vi "AB_1200_1300_Project_App_Info.vi"(6 "dataForPrevious in":T1, 7 "action":T2, 8 "error in (no error)":errorcluster, 10 "applicationInfo in":T3, 11 "Object In":T4) -> (0 "error out":errorcluster, 2 "Application info":T3, 3 "Object Out":T4, 4 "dataFromPrevious":T1)   [LabVIEW 2020]
uses:
  <resource>/Framework/Providers/API/ItemRef.ctl
  <vilib>/AppBuilder/RW_Project/AB_RW_Project_PropBag_Action.ctl
  <vilib>/AppBuilder/RW_Project/AB_RW_Project_App_Data_for_Previous.ctl
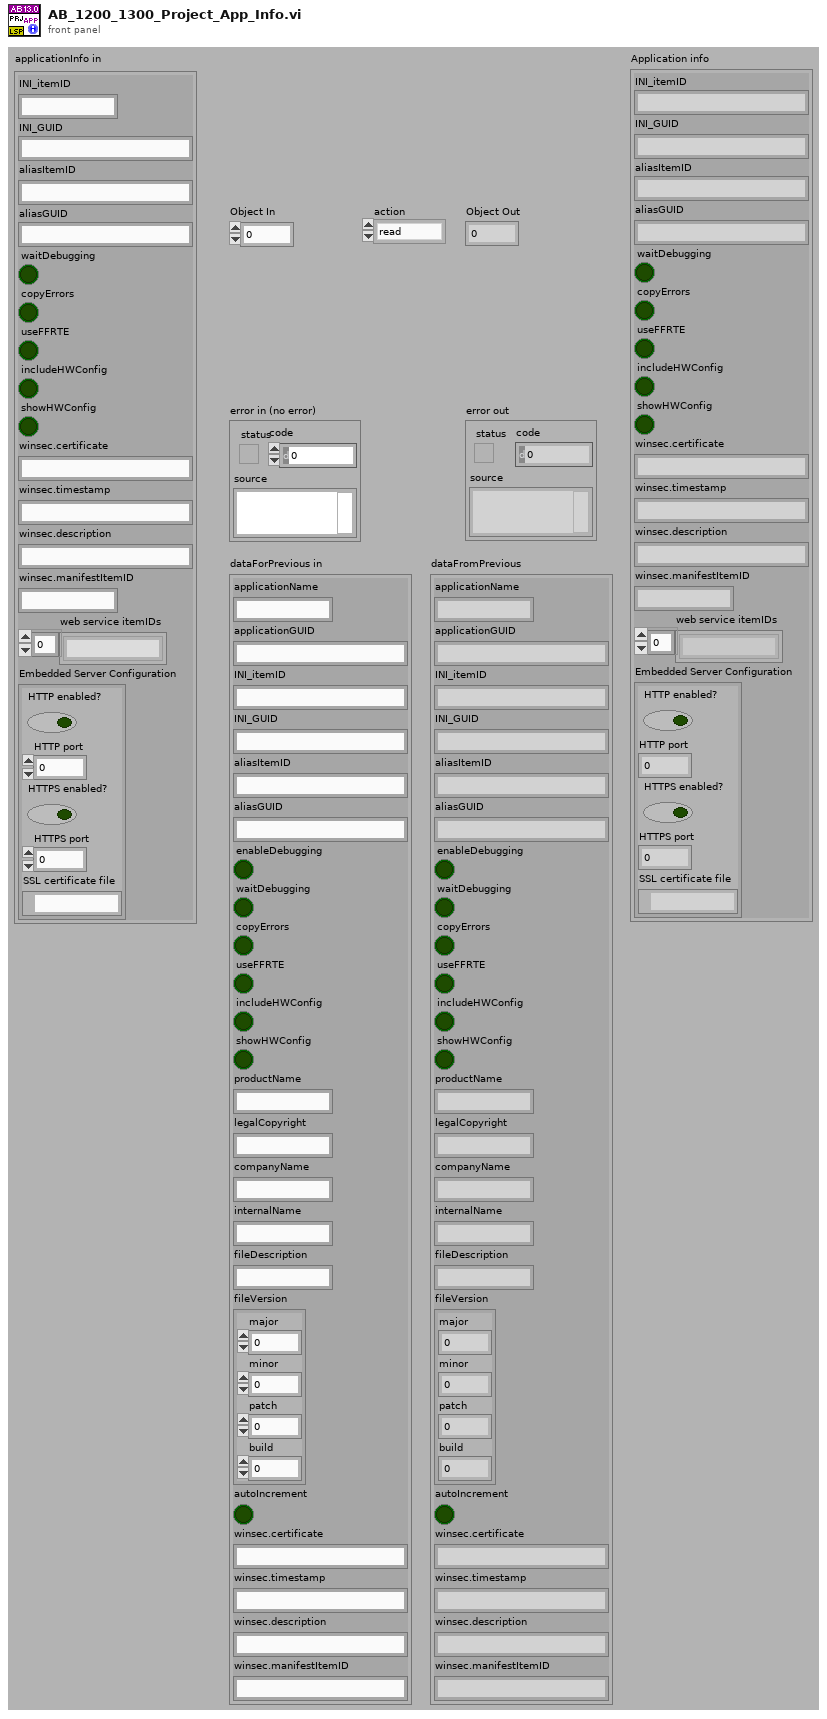
[diagram p1: front panel]
types:
  T1 = typedef "AB_RW_Project_App_Data_for_Previous.ctl" = cluster{"applicationName":string, "applicationGUID":string, "INI_itemID":string, "INI_GUID":string, "aliasItemID":string, "aliasGUID":string, "enableDebugging":bool, "waitDebugging":bool, "copyErrors":bool, "useFFRTE":bool, "includeHWConfig":bool, "showHWConfig":bool, "productName":string, "legalCopyright":string, "companyName":string, "internalName":string, "fileDescription":string, "fileVersion":cluster{"major":u16, "minor":u16, "patch":u16, "build":u16}, "autoIncrement":bool, "winsec.certificate":string, "winsec.timestamp":string, "winsec.description":string, "winsec.manifestItemID":string}
  T2 = typedef "AB_RW_Project_PropBag_Action.ctl" = enum16{"read", "write", "clear", "readPrevious", "writePrevious", "clearPrevious"}
  T3 = cluster{"INI_itemID":string, "INI_GUID":string, "aliasItemID":string, "aliasGUID":string, "waitDebugging":bool, "copyErrors":bool, "useFFRTE":bool, "includeHWConfig":bool, "showHWConfig":bool, "winsec.certificate":string, "winsec.timestamp":string, "winsec.description":string, "winsec.manifestItemID":string, "web service itemIDs":string[], "Embedded Server Configuration":cluster{"HTTP enabled?":bool, "HTTP port":i32, "HTTPS enabled?":bool, "HTTPS port":i32, "SSL certificate file":path}}
  T4 = typedef "ItemRef.ctl" = u64
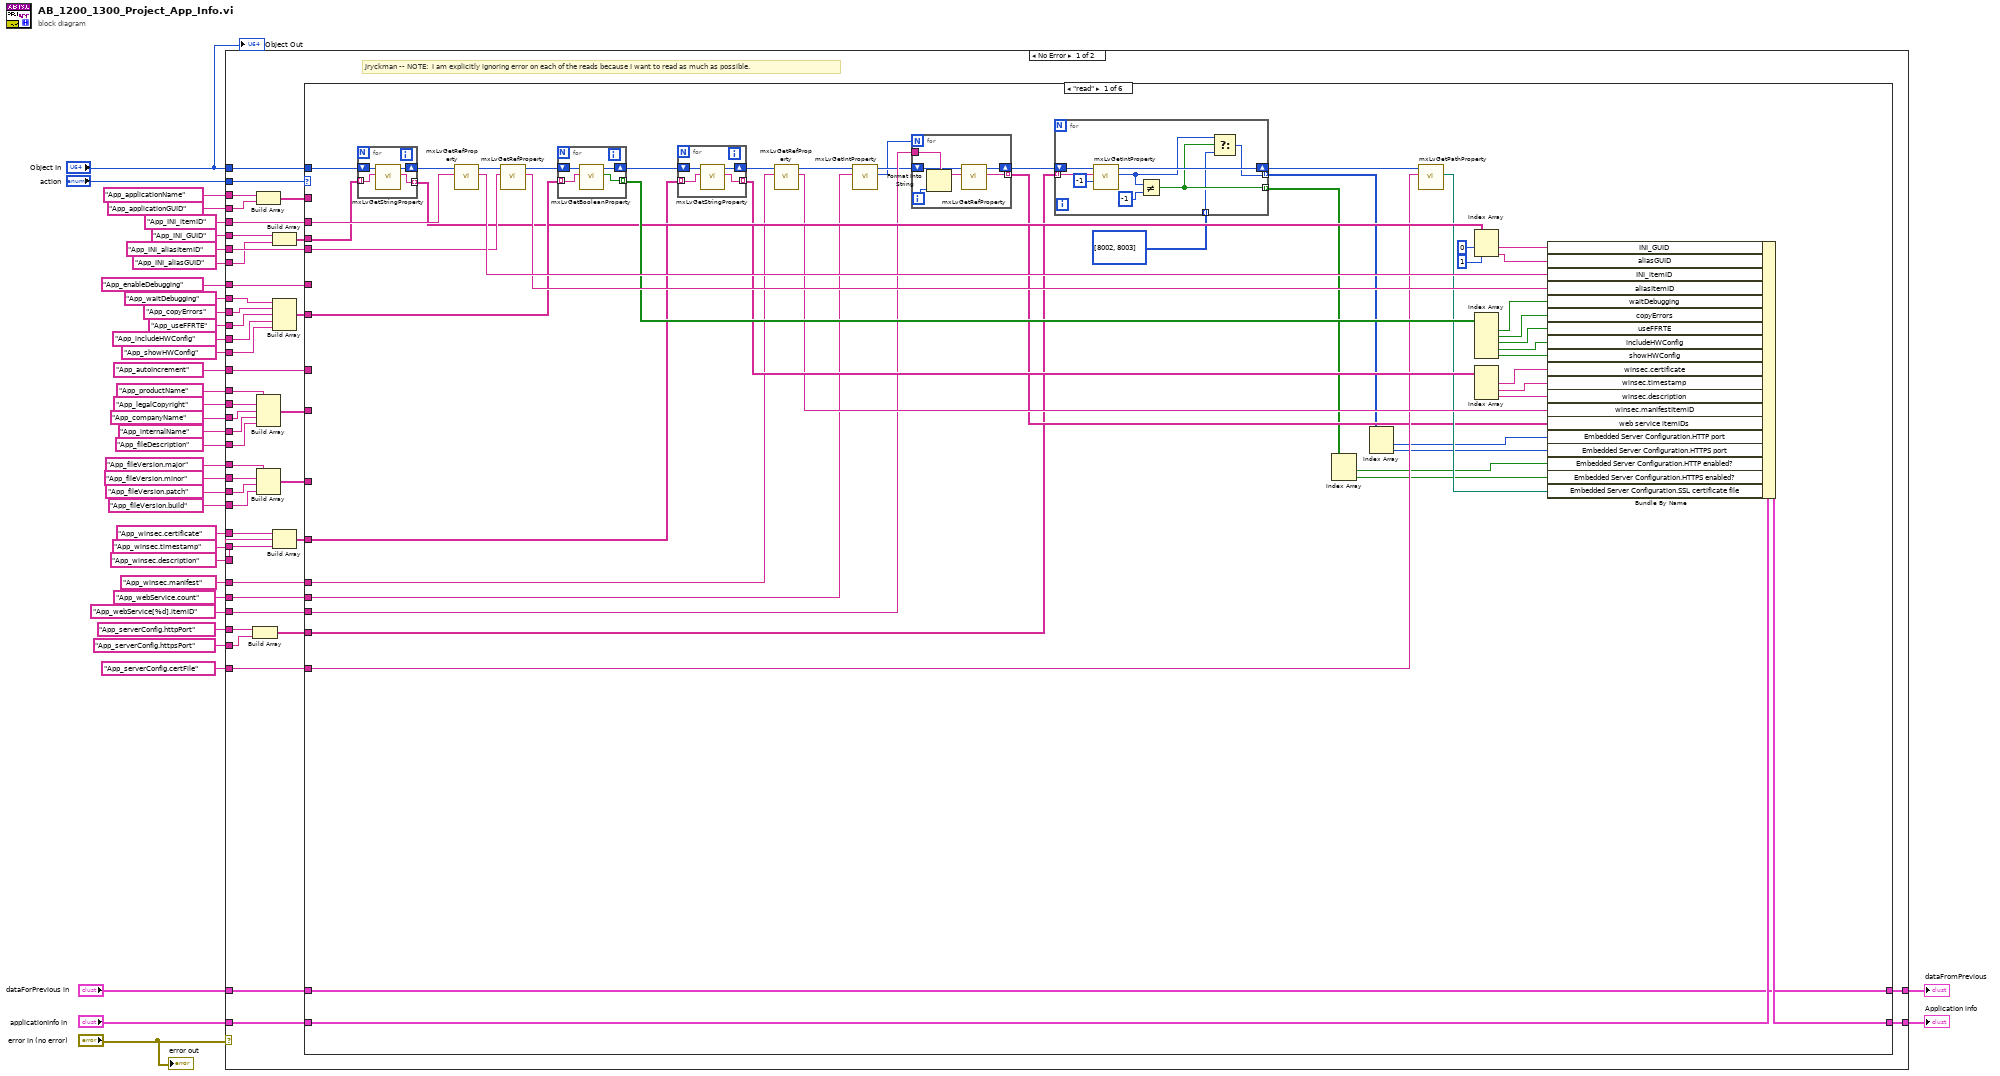
[diagram p0: block diagram]
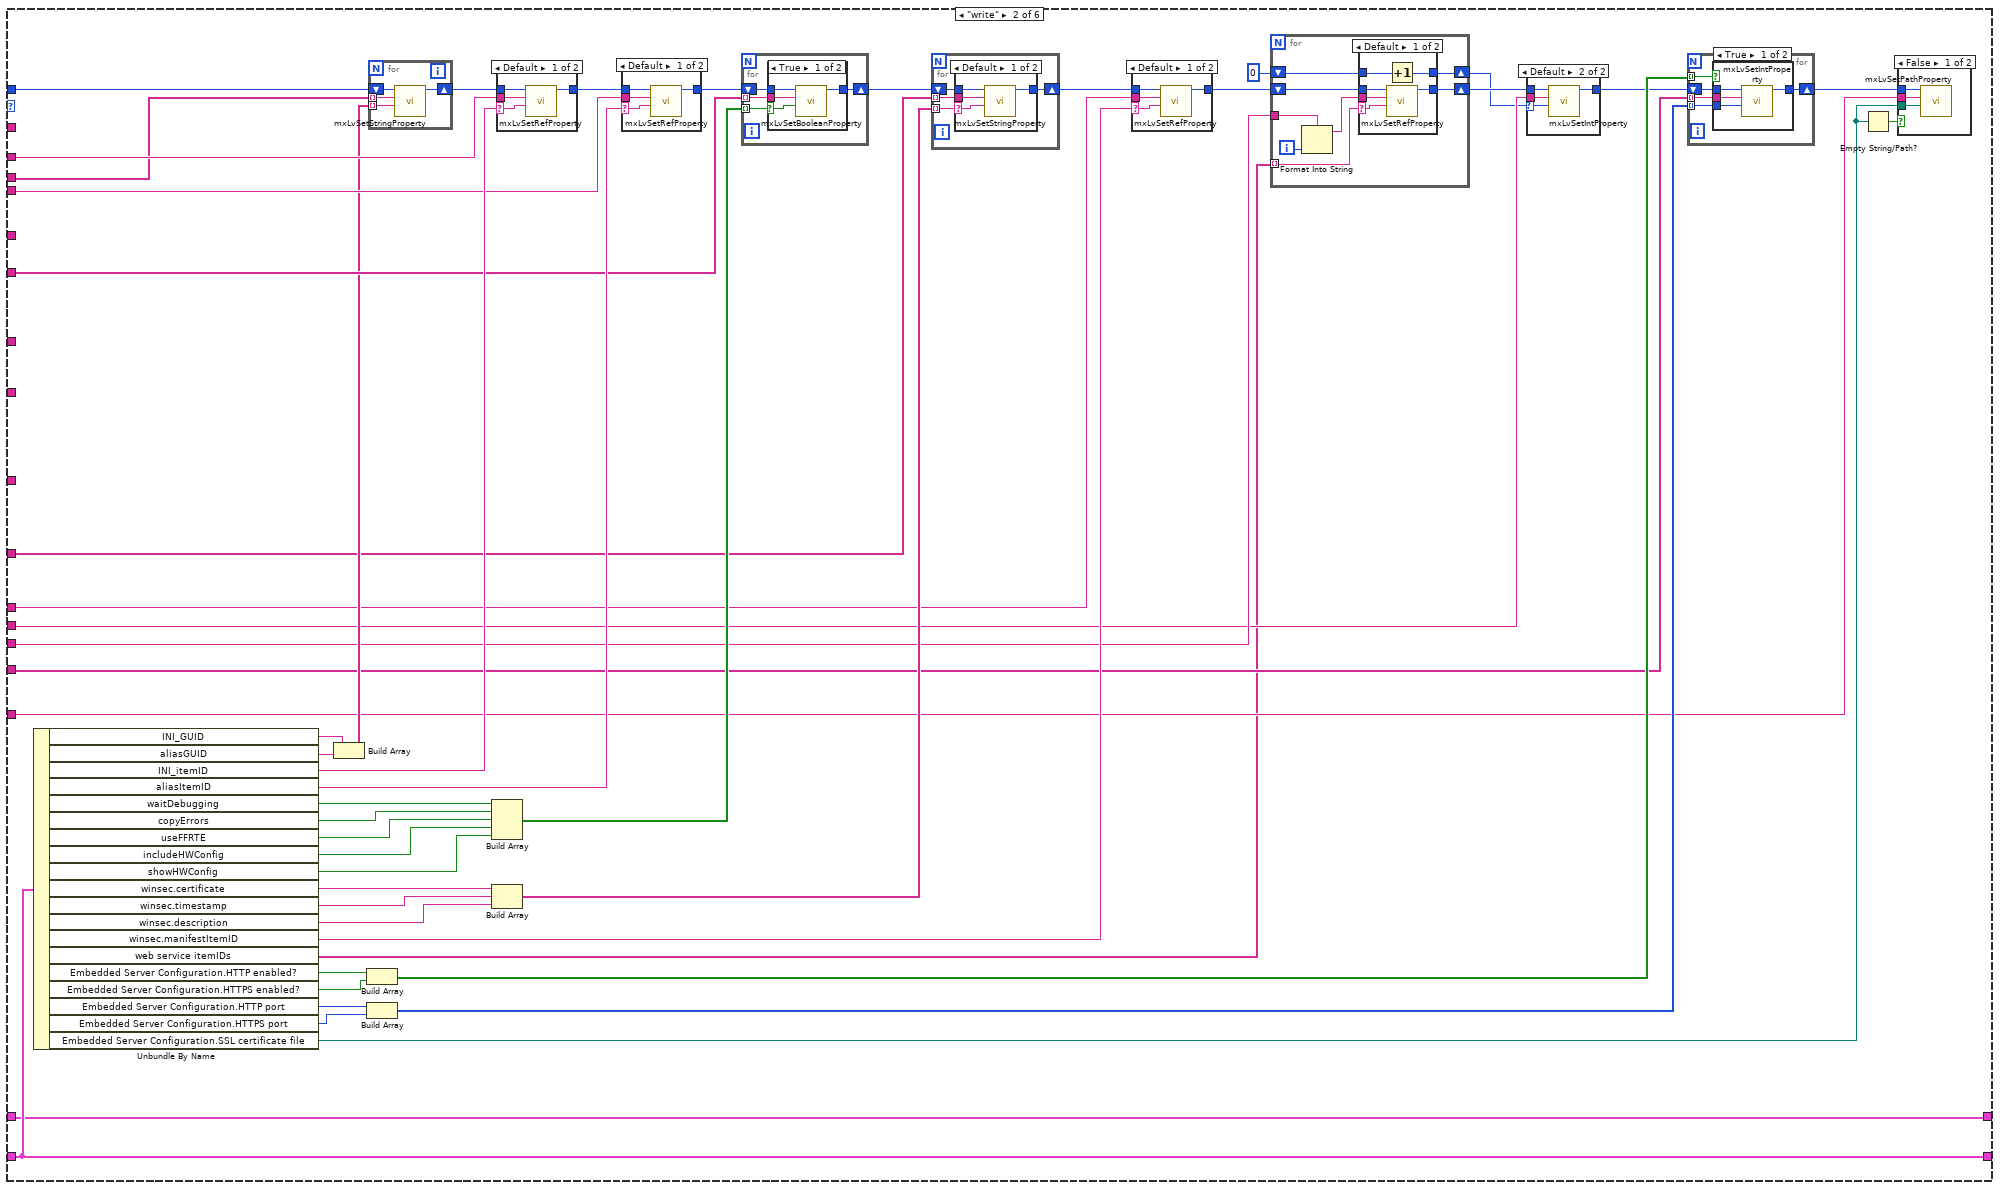
[diagram p2: hidden frame]
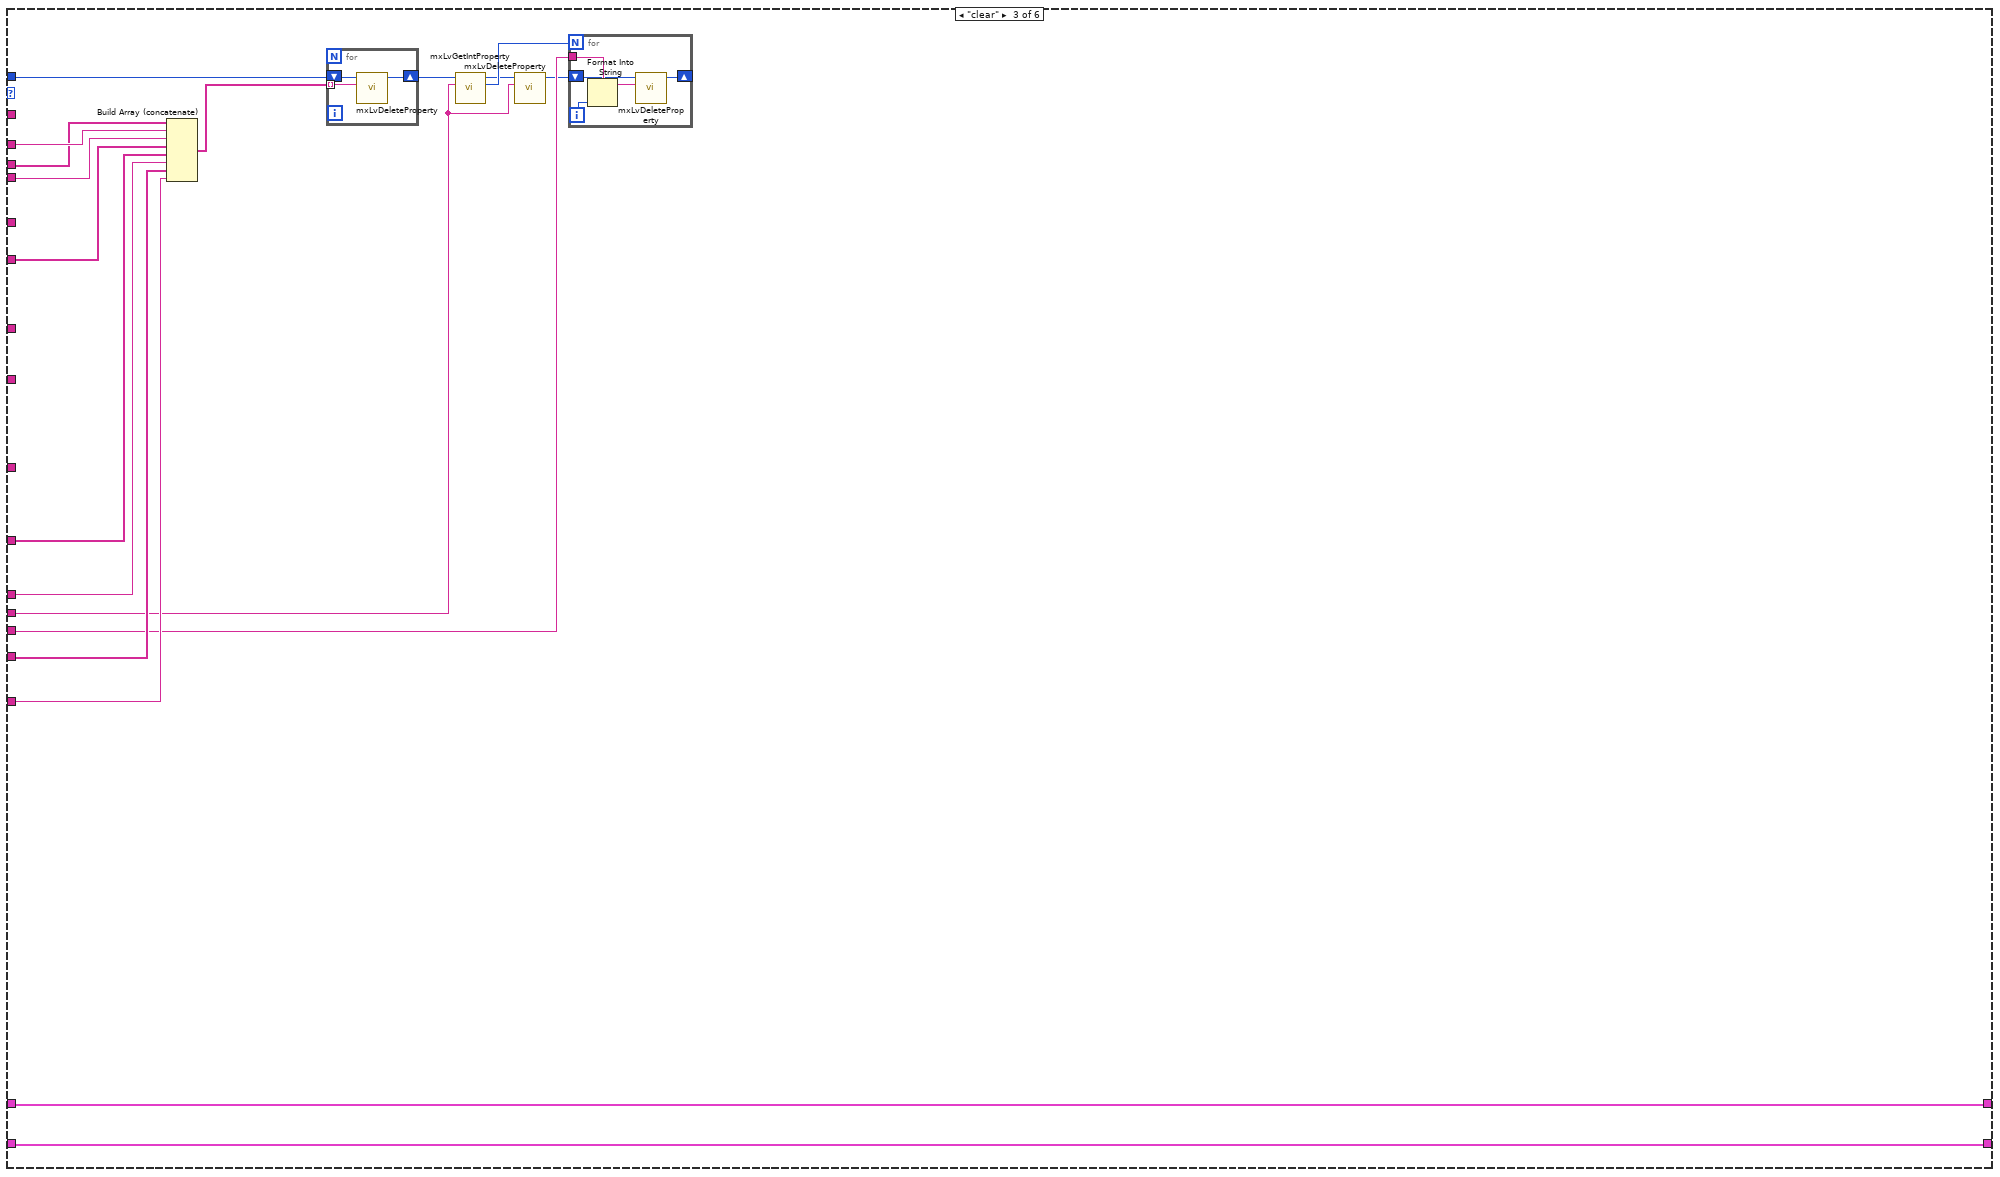
[diagram p12: hidden frame]
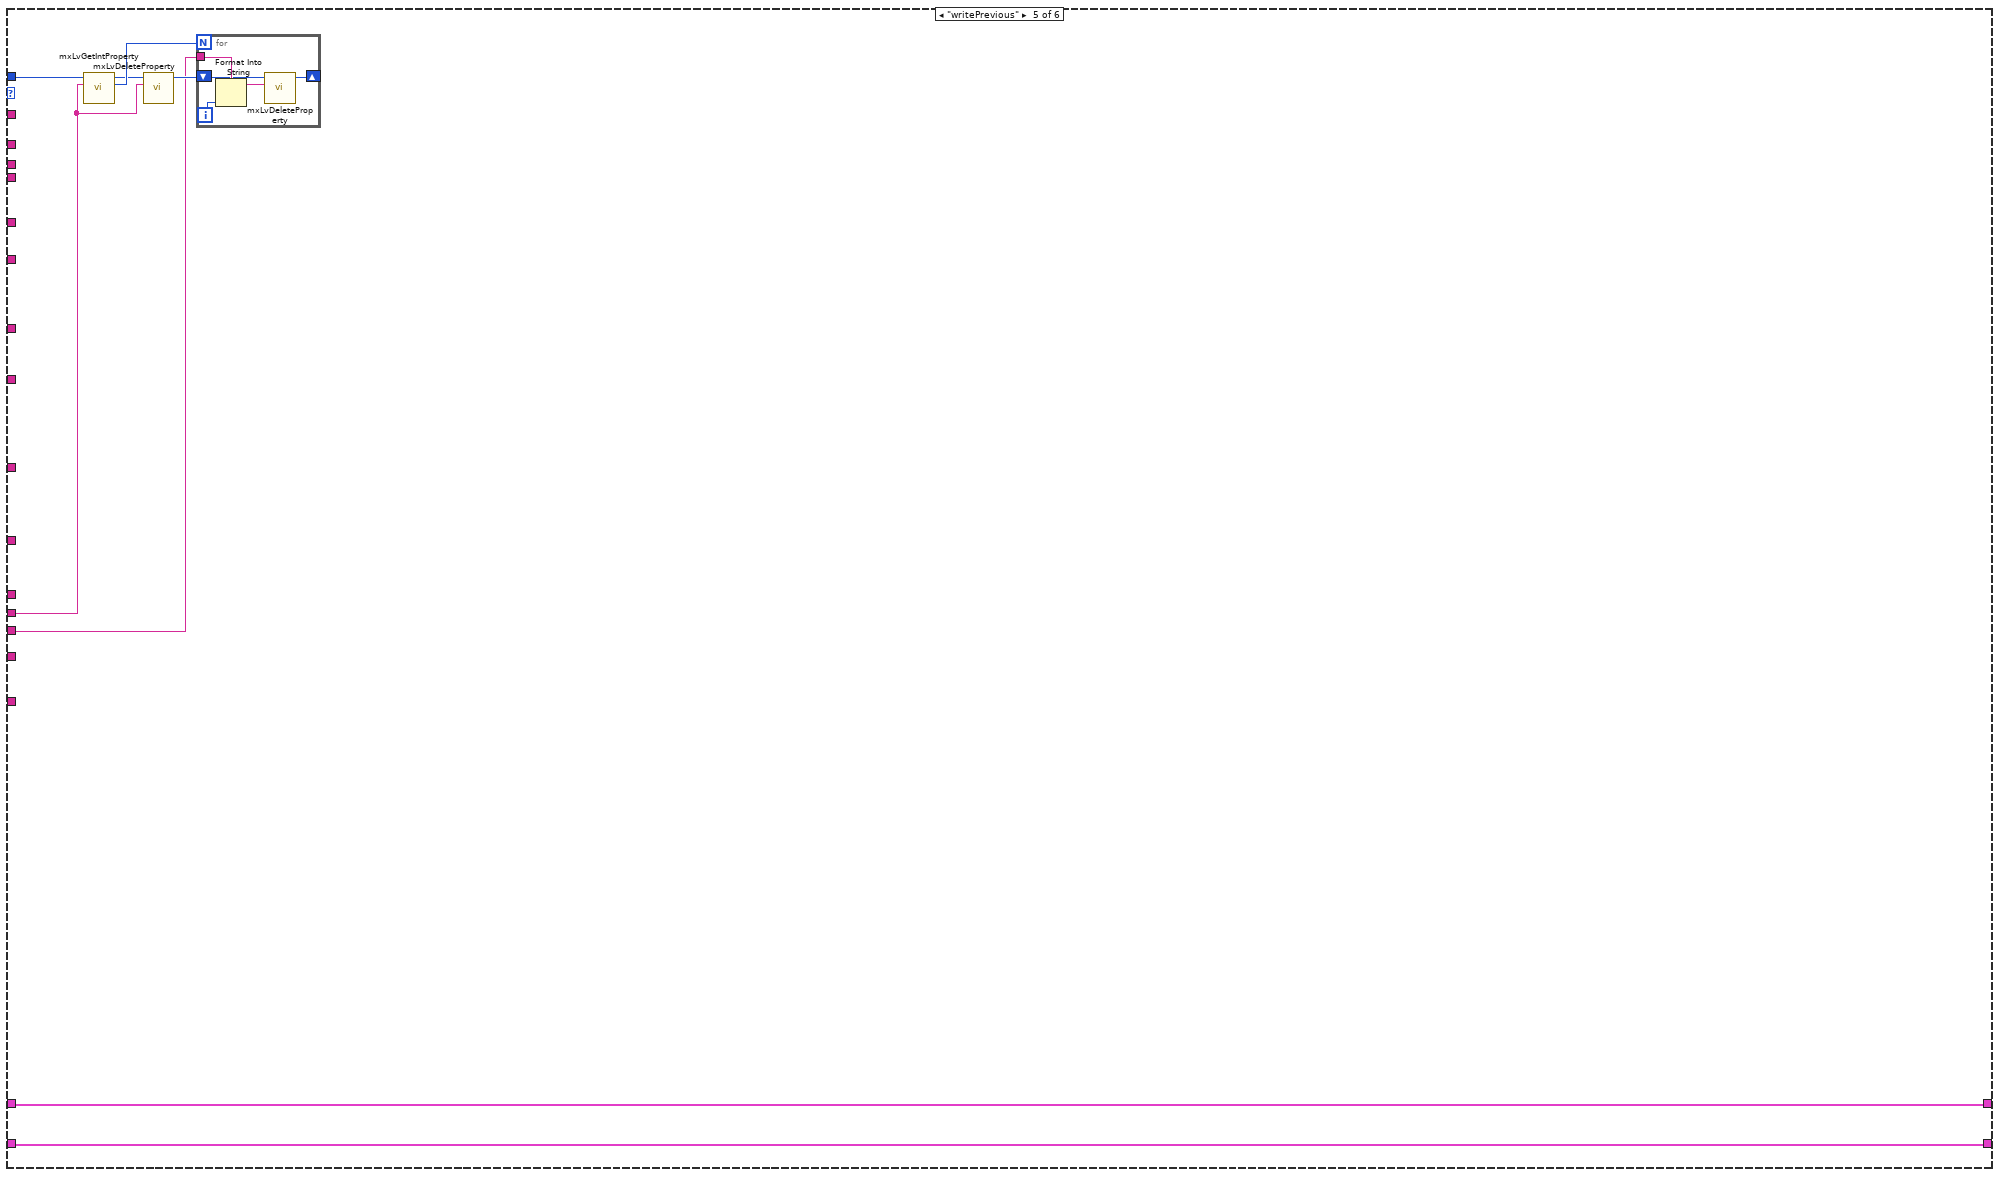
[diagram p14: hidden frame]
diagram:
  n1 = case shown="No Error" "error in (no error)" {
    tunnel: "Object In" -> [w82 _]
    tunnel: [w61 _] -> w36
    tunnel: "applicationInfo in" -> [w67 _]
    tunnel: "App_applicationName" ("Tag") -> [w48 _]
    tunnel: "App_INI_itemID" ("Tag") -> [w81 _]
    tunnel: "App_INI_aliasItemID" ("Tag") -> [w80 _]
    tunnel: "App_enableDebugging" ("Tag") -> [w50 _]
    tunnel: "App_waitDebugging" ("Tag") -> [w79 _]
    tunnel: "App_copyErrors" ("Tag") -> [w78 _]
    tunnel: "App_useFFRTE" ("Tag") -> [w77 _]
    tunnel: "App_includeHWConfig" ("Tag") -> [w76 _]
    tunnel: "App_showHWConfig" ("Tag") -> [w75 _]
    tunnel: "App_productName" ("Tag") -> [w72 _]
    tunnel: "App_legalCopyright" ("Tag") -> [w73 _]
    tunnel: "App_companyName" ("Tag") -> [w71 _]
    tunnel: "App_internalName" ("Tag") -> [w70 _]
    tunnel: "App_fileDescription" ("Tag") -> [w69 _]
    tunnel: "App_fileVersion.major" ("Tag") -> [w65 _]
    tunnel: "App_fileVersion.minor" ("Tag") -> [w66 _]
    tunnel: "App_fileVersion.patch" ("Tag") -> [w64 _]
    tunnel: "App_fileVersion.build" ("Tag") -> [w63 _]
    tunnel: "App_autoIncrement" ("Tag") -> [w49 _]
    tunnel: "action" -> [w60 _]
    tunnel: "App_applicationGUID" ("Tag") -> [w47 _]
    tunnel: "App_INI_GUID" ("Tag") -> [w59 _]
    tunnel: "App_INI_aliasGUID" ("Tag") -> [w58 _]
    tunnel: "App_winsec.certificate" ("Tag") -> [w56 _]
    tunnel: "App_winsec.timestamp" ("Tag") -> [w55 _]
    tunnel: "App_winsec.description" ("Tag") -> [w54 _]
    tunnel: "App_winsec.manifest" ("Tag") -> [w52 _]
    tunnel: "dataForPrevious in" -> [w51 _]
    tunnel: [w45 _] -> w6
    tunnel: "App_webService[%d].itemID" ("Tag") -> [w44 _]
    tunnel: "App_serverConfig.httpPort" ("Tag") -> [w43 _]
    tunnel: "App_serverConfig.httpsPort" ("Tag") -> [w42 _]
    tunnel: "App_serverConfig.certFile" ("Tag") -> [w40 _]
    tunnel: "App_webService.count" ("Tag") -> [w39 _]
    frame No Error {
      # "Jryckman -- NOTE:  I am explicitly ignoring error on each of the reads because I want to read as much as possible."
      n2 = Build Array(w43, w42) -> (w41:string[])
      n3 = Build Array(w48, w47) -> (w46:string[])
      n4 = Build Array(w72, w73, w71, w70, w69) -> (w68:string[])
      n5 = Build Array(w65, w66, w64, w63) -> (w62:string[])
      n6 = Build Array(w59, w58) -> (w57:string[])
      n7 = Build Array(w79, w78, w77, w76, w75) -> (w74:string[])
      n8 = Build Array(w56, w55, w54) -> (w53:string[])
      n9 = case shown="\"read\"" w60 {
        tunnel: w82 -> [w118 w209 w297 _ w311 _]
        tunnel: w81 -> [w129 w207 w296 _ _ _]
        tunnel: w80 -> [w128 w204 w295 _ _ _]
        tunnel: w74 -> [w126 w195 w294 _ _ _]
        tunnel: w68 -> [_ _ _ _ _ _]
        tunnel: w67 -> [w132 w194 w298 w308 w316 w323]
        tunnel: w62 -> [_ _ _ _ _ _]
        tunnel: [w119 w194 w298 w308 w316 w323] -> w61
        tunnel: w57 -> [w117 w193 w292 _ _ _]
        tunnel: w53 -> [w112 w185 w291 _ _ _]
        tunnel: w52 -> [w105 w184 w290 _ _ _]
        tunnel: w51 -> [w103 w180 w289 w307 w315 w322]
        tunnel: w50 -> [_ _ _ _ _ _]
        tunnel: w49 -> [_ _ _ _ _ _]
        tunnel: w46 -> [_ _ _ _ _ _]
        tunnel: [w103 w180 w289 w307 w315 w322] -> w45
        tunnel: w44 -> [w89 w179 w285 _ w309 _]
        tunnel: w41 -> [w94 w171 w288 _ _ _]
        tunnel: w40 -> [w97 w169 w287 _ _ _]
        tunnel: w39 -> [w85 w164 w282 _ w310 _]
        frame "read" {
          n10 = for {
            shift-right: [w155] -> w116
            shift-left: w118 -> [w156]
            tunnel: w117 -> [w153] mode=indexing
            tunnel: [w154] -> w115 mode=indexing
            n11 = call <resource>:"mxLvGetStringProperty.vi"("Tag"=w153, "Item"=w156) -> ("Value"=w154:string, "Item"=w155:T4)  [unwired: 1 in, 7 out]
          }
          n12 = call <resource>:"mxLvGetRefProperty.vi"("Tag"=w129, "Item"=w116) -> ("Value"=w131:string, "Item"=w133:T4)  [unwired: 1 in, 7 out]
          n13 = call <resource>:"mxLvGetRefProperty.vi"("Tag"=w128, "Item"=w133) -> ("Value"=w130:string, "Item"=w127:T4)  [unwired: 1 in, 7 out]
          n14 = for {
            shift-right: [w159] -> w104
            shift-left: w127 -> [w160]
            tunnel: w126 -> [w158] mode=indexing
            tunnel: [w157] -> w125 mode=indexing
            n15 = call <resource>:"mxLvGetBooleanProperty.vi"("Tag"=w158, "Item"=w160) -> ("Value"=w157:bool, "Item"=w159:T4)  [unwired: 1 in, 7 out]
          }
          n16 = for {
            shift-right: [w151] -> w107
            shift-left: w104 -> [w152]
            tunnel: w112 -> [w149] mode=indexing
            tunnel: [w150] -> w111 mode=indexing
            n17 = call <resource>:"mxLvGetStringProperty.vi"("Tag"=w149, "Item"=w152) -> ("Value"=w150:string, "Item"=w151:T4)  [unwired: 1 in, 7 out]
          }
          n18 = call <resource>:"mxLvGetRefProperty.vi"("Tag"=w105, "Item"=w107) -> ("Value"=w106:string, "Item"=w88:T4)  [unwired: 1 in, 7 out]
          n19 = call <resource>:"mxLvGetIntProperty.vi"("Tag"=w85, "Item"=w88) -> ("Value"=w86:i32, "Item"=w87:T4)  [unwired: 7 in, 1 out]
          n20 = for {
            N: w86 -> [_]
            tunnel: w89 -> [w148]
            shift-right: [w145] -> w100
            shift-left: w87 -> [w146]
            tunnel: [w144] -> w95 mode=indexing
            i -> [w147]
            n21 = Format Into String(format string=w148, w147) -> (resulting string=w143:string)  [unwired: 2 in, 1 out]
            n22 = call <resource>:"mxLvGetRefProperty.vi"("Tag"=w143, "Item"=w146) -> ("Value"=w144:string, "Item"=w145:T4)  [unwired: 7 in, 1 out]
          }
          n23 = for {
            shift-right: [w141] -> w99
            shift-left: w100 -> [w142]
            tunnel: [w135] -> w84 mode=indexing
            tunnel: w94 -> [w139] mode=indexing
            tunnel: [w137] -> w92 mode=indexing
            tunnel: i32[] [8002, 8003] -> [w134] mode=indexing
            n24 = call <resource>:"mxLvGetIntProperty.vi"("Default Value (0)"=-1, "Tag"=w139, "Item"=w142) -> ("Value"=w136:i32, "Item"=w141:T4)  [unwired: 6 in, 1 out]
            n25 = Not Equal?(x=w136, y=-1 ("Default Value (0)")) -> (x != y?=w137:bool)
            n26 = Select(t=w136, s=w137, f=w134) -> (s? t:f=w135:i32)
          }
          n27 = Index Array(array=w92) -> (element #1=w91:bool, element #2=w90:bool)  [unwired: 2 in]
          n28 = Index Array(array=w84) -> (element #1=w93:i32, element #2=w96:i32)  [unwired: 2 in]
          n29 = call <resource>:"mxLvGetPathProperty.vi"("Tag"=w97, "Item"=w99) -> ("Path"=w98:path)  [unwired: 7 in, 2 out]
          n30 = Index Array(array=w115, index #1=0 ("index"), index #2=1 ("index")) -> (element #1=w114:string, element #2=w113:string)
          n31 = Index Array(array=w125) -> (element #1=w124:bool, element #2=w123:bool, element #3=w122:bool, element #4=w121:bool, element #5=w120:bool)  [unwired: 5 in]
          n32 = Index Array(array=w111) -> (element #1=w110:string, element #2=w109:string, element #3=w108:string)  [unwired: 3 in]
          n33 = Bundle By Name(cluster=w132, "INI_GUID"=w114, "aliasGUID"=w113, "INI_itemID"=w131, "aliasItemID"=w130, "waitDebugging"=w124, "copyErrors"=w123, "useFFRTE"=w122, "includeHWConfig"=w121, "showHWConfig"=w120, "winsec.certificate"=w110, "winsec.timestamp"=w109, "winsec.description"=w108, "winsec.manifestItemID"=w106, "web service itemIDs"=w95, "Embedded Server Configuration.HTTP port"=w93, "Embedded Server Configuration.HTTPS port"=w96, "Embedded Server Configuration.HTTP enabled?"=w91, "Embedded Server Configuration.HTTPS enabled?"=w90, "Embedded Server Configuration.SSL certificate file"=w98) -> (w119:T3)
        }
        frame "write" {
          n34 = Unbundle By Name(w194) -> ("INI_GUID"=w190:string, "aliasGUID"=w192:string, "INI_itemID"=w206:string, "aliasItemID"=w203:string, "waitDebugging"=w201:bool, "copyErrors"=w200:bool, "useFFRTE"=w199:bool, "includeHWConfig"=w198:bool, "showHWConfig"=w197:bool, "winsec.certificate"=w189:string, "winsec.timestamp"=w188:string, "winsec.description"=w187:string, "winsec.manifestItemID"=w182:string, "web service itemIDs"=w163:string[], "Embedded Server Configuration.HTTP enabled?"=w177:bool, "Embedded Server Configuration.HTTPS enabled?"=w176:bool, "Embedded Server Configuration.HTTP port"=w175:i32, "Embedded Server Configuration.HTTPS port"=w174:i32, "Embedded Server Configuration.SSL certificate file"=w168:path)
          n35 = Build Array(w190, w192) -> (w191:string[])
          n36 = Build Array(w177, w176) -> (w173:bool[])
          n37 = Build Array(w175, w174) -> (w172:i32[])
          n38 = for {
            tunnel: w193 -> [w259] mode=indexing
            tunnel: w191 -> [w258] mode=indexing
            shift-right: [w260] -> w208
            shift-left: w209 -> [w261]
            n39 = call <resource>:"mxLvSetStringProperty.vi"("Value (\"\")"=w258, "Tag"=w259, "Item"=w261) -> ("Item"=w260:T4)  [unwired: 2 in, 6 out]
          }
          n40 = Build Array(w201, w200, w199, w198, w197) -> (w196:bool[])
          n41 = Build Array(w189, w188, w187) -> (w186:string[])
          n42 = case shown="Default" w206 {
            selector: w206 -> [w277 _]
            tunnel: w208 -> [w279 w280]
            tunnel: w207 -> [w278 _]
            tunnel: [w276 w280] -> w205
            frame Default {
              n43 = call <resource>:"mxLvSetRefProperty.vi"("Value (\"\")"=w277, "Tag"=w278, "Item"=w279) -> ("Item"=w276:T4)  [unwired: 2 in, 6 out]
            }
            frame "" {
            }
          }
          n44 = case shown="Default" w203 {
            selector: w203 -> [w272 _]
            tunnel: w205 -> [w274 w275]
            tunnel: w204 -> [w273 _]
            tunnel: [w271 w275] -> w202
            frame Default {
              n45 = call <resource>:"mxLvSetRefProperty.vi"("Value (\"\")"=w272, "Tag"=w273, "Item"=w274) -> ("Item"=w271:T4)  [unwired: 2 in, 6 out]
            }
            frame "" {
            }
          }
          n46 = for {
            tunnel: w196 -> [w264] mode=indexing
            shift-right: [w263] -> w181
            shift-left: w202 -> [w265]
            tunnel: w195 -> [w262] mode=indexing
            n47 = case shown="True" w264 {
              selector: w264 -> [w268 _]
              tunnel: w265 -> [w269 w270]
              tunnel: w262 -> [w266 _]
              tunnel: [w267 w270] -> w263
              frame True {
                n48 = call <resource>:"mxLvSetBooleanProperty.vi"("Value (F)"=w268, "Tag"=w266, "Item"=w269) -> ("Item"=w267:T4)  [unwired: 2 in, 6 out]
              }
              frame False {
              }
            }
          }
          n49 = for {
            tunnel: w186 -> [w251] mode=indexing
            shift-right: [w250] -> w183
            shift-left: w181 -> [w252]
            tunnel: w185 -> [w249] mode=indexing
            n50 = case shown="Default" w251 {
              selector: w251 -> [w254 _]
              tunnel: w252 -> [w256 w257]
              tunnel: w249 -> [w253 _]
              tunnel: [w255 w257] -> w250
              frame Default {
                n51 = call <resource>:"mxLvSetStringProperty.vi"("Value (\"\")"=w254, "Tag"=w253, "Item"=w256) -> ("Item"=w255:T4)  [unwired: 2 in, 6 out]
              }
              frame "" {
              }
            }
          }
          n52 = case shown="Default" w182 {
            selector: w182 -> [w245 _]
            tunnel: w183 -> [w247 w248]
            tunnel: w184 -> [w246 _]
            tunnel: [w244 w248] -> w178
            frame Default {
              n53 = call <resource>:"mxLvSetRefProperty.vi"("Value (\"\")"=w245, "Tag"=w246, "Item"=w247) -> ("Item"=w244:T4)  [unwired: 2 in, 6 out]
            }
            frame "" {
            }
          }
          n54 = for {
            tunnel: w179 -> [w235]
            tunnel: w163 -> [w233] mode=indexing
            shift-right: [w231] -> w166
            shift-left: w178 -> [w232]
            shift-right: [w228] -> w161
            shift-left: 0 -> [w229]
            i -> [w234]
            n55 = Format Into String(format string=w235, w234) -> (resulting string=w230:string)  [unwired: 2 in, 1 out]
            n56 = case shown="Default" w233 {
              selector: w233 -> [w236 _]
              tunnel: w232 -> [w239 w243]
              tunnel: w230 -> [w237 _]
              tunnel: [w238 w243] -> w231
              tunnel: w229 -> [w241 w242]
              tunnel: [w240 w242] -> w228
              frame Default {
                n57 = Increment(x=w241) -> (x+1=w240:i32)
                n58 = call <resource>:"mxLvSetRefProperty.vi"("Value (\"\")"=w236, "Tag"=w237, "Item"=w239) -> ("Item"=w238:T4)  [unwired: 7 in, 1 out]
              }
              frame "" {
              }
            }
          }
          n59 = case shown="Default" w161 {
            selector: w161 -> [_ w212]
            tunnel: w166 -> [w210 w214]
            tunnel: [w210 w213] -> w165
            tunnel: w164 -> [_ w211]
            frame 0 {
            }
            frame Default {
              n60 = call <resource>:"mxLvSetIntProperty.vi"("Value (0)"=w212, "Tag"=w211, "Item"=w214) -> ("Item"=w213:T4)  [unwired: 7 in, 1 out]
            }
          }
          n61 = for {
            tunnel: w173 -> [w221] mode=indexing
            shift-right: [w220] -> w170
            shift-left: w165 -> [w222]
            tunnel: w172 -> [w219] mode=indexing
            tunnel: w171 -> [w218] mode=indexing
            n62 = case shown="True" w221 {
              tunnel: w222 -> [w226 w227]
              tunnel: w219 -> [w224 _]
              tunnel: [w225 w227] -> w220
              tunnel: w218 -> [w223 _]
              frame True {
                n63 = call <resource>:"mxLvSetIntProperty.vi"("Value (0)"=w224, "Tag"=w223, "Item"=w226) -> ("Item"=w225:T4)  [unwired: 7 in, 1 out]
              }
              frame False {
              }
            }
          }
          n64 = Empty String/Path?(string/path=w168) -> (empty?=w167:bool)
          n65 = case shown="False" w167 {
            tunnel: w170 -> [w217 _]
            tunnel: w169 -> [w216 _]
            tunnel: w168 -> [w215 _]
            frame False {
              n66 = call <resource>:"mxLvSetPathProperty.vi"("Path"=w215, "Tag"=w216, "Item"=w217) -> ()  [unwired: 7 in, 2 out]
            }
            frame True {
            }
          }
        }
        frame "clear" {
          n67 = Build Array (concatenate)(w292, w296, w295, w294, w291, w290, w288, w287) -> (w293:string[])
          n68 = for {
            tunnel: w293 -> [w305] mode=indexing
            shift-right: [w304] -> w281
            shift-left: w297 -> [w306]
            n69 = call <resource>:"mxLvDeleteProperty.vi"("Tag"=w305, "Item"=w306) -> ("Item"=w304:T4)  [unwired: 1 in, 8 out]
          }
          n70 = call <resource>:"mxLvGetIntProperty.vi"("Tag"=w282, "Item"=w281) -> ("Value"=w286:i32, "Item"=w284:T4)  [unwired: 7 in, 1 out]
          n71 = call <resource>:"mxLvDeleteProperty.vi"("Tag"=w282, "Item"=w284) -> ("Item"=w283:T4)  [unwired: 1 in, 8 out]
          n72 = for {
            N: w286 -> [_]
            tunnel: w285 -> [w303]
            shift-right: [w299] -> _
            shift-left: w283 -> [w301]
            i -> [w302]
            n73 = Format Into String(format string=w303, w302) -> (resulting string=w300:string)  [unwired: 2 in, 1 out]
            n74 = call <resource>:"mxLvDeleteProperty.vi"("Tag"=w300, "Item"=w301) -> ("Item"=w299:T4)  [unwired: 1 in, 8 out]
          }
        }
        frame "readPrevious" {
        }
        frame "writePrevious" {
          n75 = call <resource>:"mxLvGetIntProperty.vi"("Tag"=w310, "Item"=w311) -> ("Value"=w314:i32, "Item"=w313:T4)  [unwired: 7 in, 1 out]
          n76 = call <resource>:"mxLvDeleteProperty.vi"("Tag"=w310, "Item"=w313) -> ("Item"=w312:T4)  [unwired: 1 in, 8 out]
          n77 = for {
            N: w314 -> [_]
            tunnel: w309 -> [w321]
            shift-right: [w317] -> _
            shift-left: w312 -> [w319]
            i -> [w320]
            n78 = Format Into String(format string=w321, w320) -> (resulting string=w318:string)  [unwired: 2 in, 1 out]
            n79 = call <resource>:"mxLvDeleteProperty.vi"("Tag"=w318, "Item"=w319) -> ("Item"=w317:T4)  [unwired: 1 in, 8 out]
          }
        }
        frame "clearPrevious" {
        }
      }
    }
    frame Error {
    }
  }
  "Application info" <- w36
  "dataFromPrevious" <- w6
  "Object Out" <- "Object In"
  "error out" <- "error in (no error)"
